vi "TCP_read_string.vi"(8 "error in (no error)":errorcluster, 11 "TCP Network Connection in":refnum<k5>) -> (0 "error out":errorcluster, 2 "output":string, 3 "TCP Network Connection out":refnum<k5>)   [LabVIEW 2017]
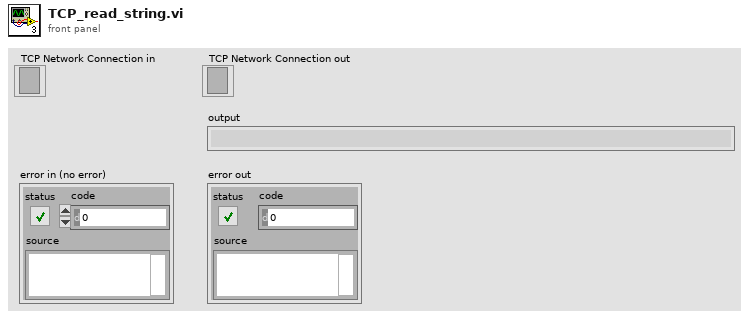
[diagram p1: front panel]
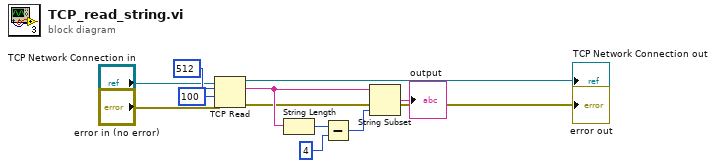
[diagram p0: block diagram]
diagram:
  n1 = TCP Read(connection ID="TCP Network Connection in", bytes to read=512, error in (no error)="error in (no error)", 9:100 ("timeout ms (25000)")) -> (connection ID out=→"TCP Network Connection out":refnum<k5>, data out=w7:string, error out=→"error out":errorcluster)  [unwired: 1 in]
  n2 = String Length(string=w7) -> (length=w8:i32)
  n3 = Subtract(x=w8, y=4) -> (x-y=w10:i32)
  n4 = String Subset(string=w7, length (rest)=w10) -> (substring=→"output":string)  [unwired: 1 in]
